vi "servo analog(SubVI).vi"(6 "Offset":dbl=2.5, 7 "Duty Cycle (%)":dbl(slide)=50.0 scale=0.0..150.0, 9 "Amplitude":dbl=2.5, 10 "Frequency":dbl=50.0, 11 "stop (F)":bool) -> (2 "Square":dynamicdata(graph), 3 "stopped":bool)   [LabVIEW 2022 SP3]
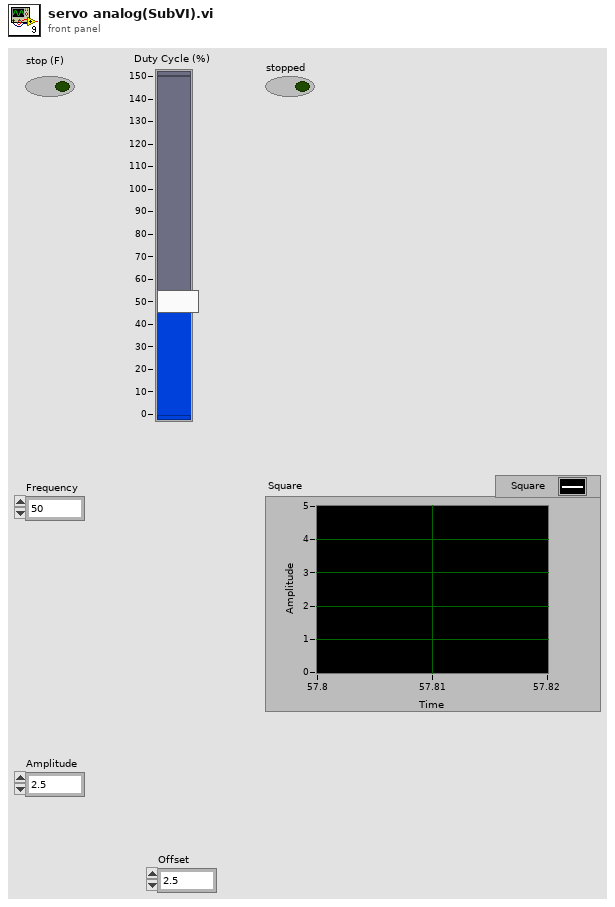
[diagram p1: front panel]
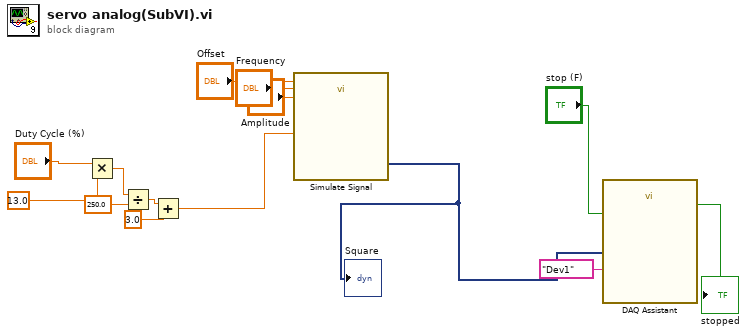
[diagram p0: block diagram]
diagram:
  n1 = Multiply(x="Duty Cycle (%)", y=13.0) -> (x*y=w8:dbl)
  n2 = Divide(x=w8, y=250.0) -> (x/y=w9:dbl)
  n3 = Add(x=w9, y=3.0) -> (x+y=w14:dbl)
  n4 = call "Simulate Signal"("Offset"="Offset", "Duty Cycle (%)"=w14, "Frequency"="Frequency", "Amplitude"="Amplitude") -> ("Square"=w6:dynamicdata)  [unwired: 10 in, 1 out]
  "Square" <- w6
  n5 = call "DAQ Assistant"("data"=w6, "stop (F)"="stop (F)", "device name"=tag "Dev1") -> ("stopped"=→"stopped":bool)  [unwired: 14 in, 2 out]
